vi "Print Function Description.vi"(10 "functionDescription":string, 11 "functionName":string) -> (2 "functionDescription out":string, 3 "functionName out":string)   [LabVIEW 2018, in "ParsingDataSampleDLL.lvlib"]
doc: "__declspec(dllexport) void PrintFunctionDescription(char *functionName, char *functionDescription);"
uses:
  ParsingDataSampleDLL.lvlib
  ni_reference_vs/Debug/ParsingDataSampleDLL.dll
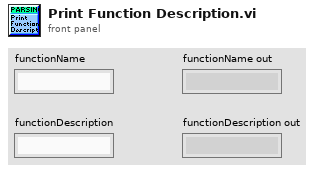
[diagram p1: front panel]
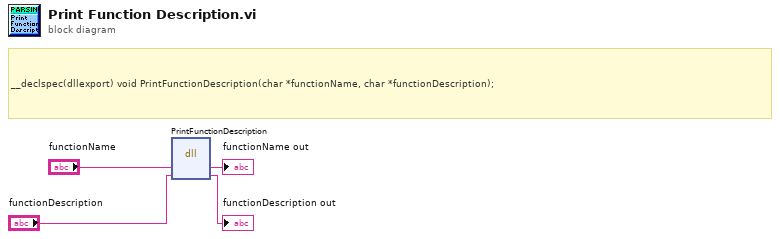
[diagram p0: block diagram]
diagram:
  # "__declspec(dllexport) void PrintFunctionDescription(char *functionName, char *functionDescription);"
  n1 = dll-call lib="C:/Users/celit/Documents/GitHub/Labview_Python_DLL_Call/ni_reference_vs/Debug/ParsingDataSampleDLL.*" fn="PrintFunctionDescription"("functionName"="functionName", "functionDescription"="functionDescription") -> ("functionName"=→"functionName out":string, "functionDescription"=→"functionDescription out":string)  [unwired: 4 in, 2 out]
